vi "Get Path.vi"(1 "path":path, 2 "Event Name":string, 3 "OK Button":bool) -> (0 "Event Location":string)   [LabVIEW 2014]
panel:
  out "string":string
  out "filenames":string[](array[string])
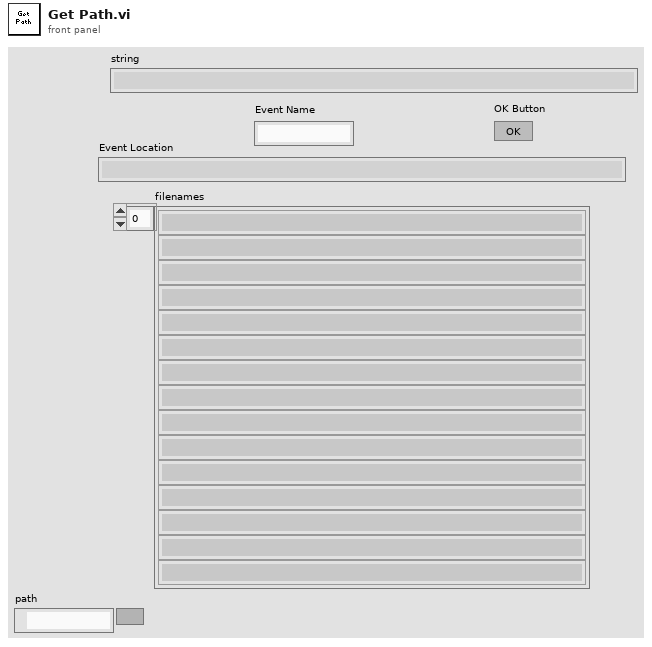
[diagram p1: front panel]
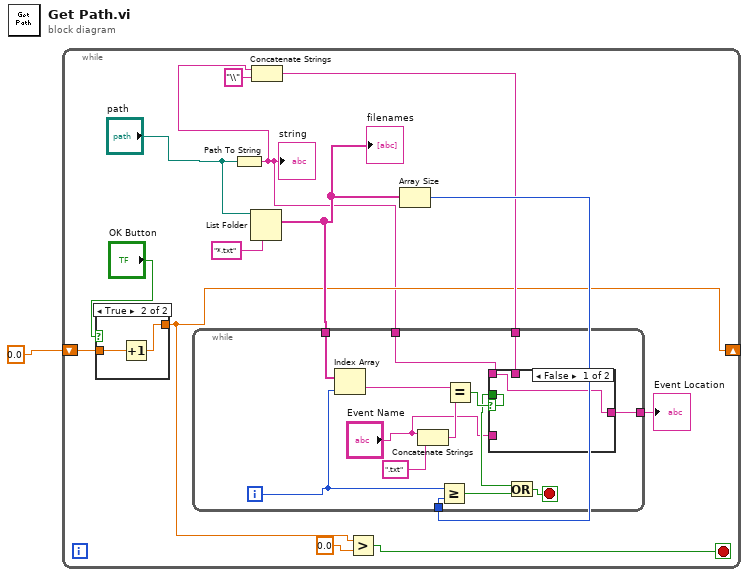
[diagram p0: block diagram]
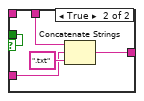
[diagram p3: hidden frame]
diagram:
  n1 = while {
    shift-right: [w5] -> _
    shift-left: 0.0 ("Numeric") -> [w7]
    stop <- w4 stop-if-true
    n2 = case shown="True" "OK Button" {
      tunnel: w7 -> [w15 w17]
      tunnel: [w15 w16] -> w5
      frame False {
      }
      frame True {
        n3 = Increment(x=w17) -> (x+1=w16:dbl)
      }
    }
    n4 = Path To String(path="path") -> (string=w3:string)
    "string" <- w3
    n5 = List Folder(path="path", pattern="*.txt") -> (filenames=w13:string[])  [unwired: 2 in, 3 out]
    "filenames" <- w13
    n6 = Concatenate Strings(w3, "\\" ("string")) -> (w10:string)
    n7 = Greater?(x=w5, y=0.0) -> (0:w4:bool)
    n8 = Array Size(array=w13) -> (size(s)=w12:i32)
    n9 = while {
      tunnel: w13 -> [w31]
      tunnel: w12 -> [w27]
      tunnel: w10 -> [w24]
      tunnel: [w23] -> w9
      tunnel: w3 -> [w19]
      i -> [w28]
      stop <- w30 stop-if-true
      n10 = Index Array(array=w31, index=w28) -> (element=w26:string)
      n11 = Concatenate Strings("Event Name", ".txt" ("string")) -> (w21:string)
      n12 = Greater Or Equal?(x=w28, y=w27) -> (x >= y?=w29:bool)
      n13 = Equal?(x=w26, y=w21) -> (x = y?=w25:bool)
      n14 = case shown="False" w25 {
        selector: w25 -> [w33 w35]
        tunnel: w24 -> [_ w38]
        tunnel: [w32 w36] -> w23
        tunnel: [w33 w35] -> w22
        tunnel: "Event Name" -> [_ w34]
        tunnel: w19 -> [w32 _]
        frame False {
        }
        frame True {
          n15 = Concatenate Strings(w38, w34, ".txt" ("string")) -> (w36:string)
        }
      }
      n16 = Or(x=w22, y=w29) -> (x .or. y?=w30:bool)
    }
    "Event Location" <- w9
  }
